vi "tools_openWebPage.vi"   [LabVIEW 2023]
uses:
  <vilib>/Platform/browser.llb/Open URL in Default Browser (string).vi
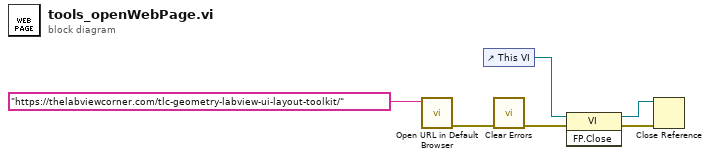
[diagram p0: block diagram]
diagram:
  n1 = call-poly <vilib>:"Open URL in Default Browser.vi"("URL"="https://thelabviewcorner.com/tlc-geometry-labview-ui-layout-toolkit/") -> ("error out"=w2:errorcluster)  [unwired: 5 in, 1 out]
  n2 = control-ref of="This VI"() -> (w6:refnum<vi>)
  n3 = call <vilib>:"Clear Errors.vi"("error in (no error)"=w2) -> ("error out"=w3:errorcluster)  [unwired: 5 in, 1 out]
  n4 = invoke class="VI" method="FP.Close"(reference=w6, error in=w3) -> (reference out=w5:refnum<vi>, error out=w4:errorcluster)  [unwired: 1 in, 1 out]
  n5 = Close Reference(reference=w5, error in (no error)=w4) -> ()  [unwired: 1 out]
